vi "test Check UDP Properties and Redundancy.vi"(8 "error in":errorcluster, 11 "TestCase in":refnum<class "AIM ARINC 664 EncodeDecode.lvclass">) -> (0 "error out":errorcluster, 3 "TestCase out":refnum<class "AIM ARINC 664 EncodeDecode.lvclass">)   [LabVIEW 2020, in "AIM ARINC 664 EncodeDecode.lvclass"]
uses:
  AIM ARINC 664 EncodeDecode.lvclass
  C:/Program Files (x86)/National Instruments/LabVIEW 2020/vi.lib/NI/VeriStand Custom Device Testing Tools/VeriStandScriptingTestCase/VeriStandScriptingTestCase.lvclass
  Import/_typedefs/board_setup.ctl
  Import/_typedefs/tx_udp_setup.ctl
  Import/_typedefs/port_tx_udp_comm.ctl
  Import/_typedefs/frame_parameter.ctl
  Import/_typedefs/frame_parameter_definition.ctl
  <vilib>/NI/NI VeriStand Encoding and Decoding/Encoding.ctl
  Import/_typedefs/port_tx_udp_sap.ctl
  Import/_typedefs/rx_udp_setup.ctl
  Import/_typedefs/port_rx_udp_comm.ctl
  Import/_typedefs/port_rx_udp_sap.ctl
  <vilib>/NI/VeriStand Custom Device Testing Tools/VeriStandScriptingTestCase/VeriStandScriptingTestCase.lvclass/VeriStandScriptingTestCase.ctl
  <vilib>/NI/VeriStand Custom Device Testing Tools/VeriStandScriptingTestCase/Read Target.vi
  NationalInstruments.VeriStand.SystemDefinitionAPI
  <vilib>/addons/_JKI Toolkits/VI Tester/TestCase.llb/TestCase.lvclass
  Scripting/AIM ARINC 664 Scripting.lvlib
  Import/AIM ARINC 664 Import.lvlib
  <vilib>/NI/NI VeriStand Encoding and Decoding/Encoding and Decoding.lvlib
  C:/Program Files (x86)/National Instruments/LabVIEW 2020/vi.lib/addons/_JKI Toolkits/VI Tester/TestCase.llb/TestCase.lvclass
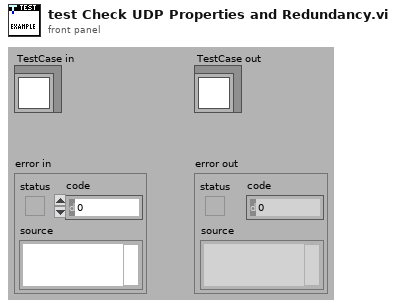
[diagram p1: front panel]
types:
  T1 = typedef "AIM ARINC 664 Import.lvlib/rx_udp_setup.ctl" = cluster{"VerificationMode":u32, "Bag":u32, "Jitter":u32, "MaxFrameLength":u32, "MaxSkew":u32, "VLBufSize":u32, "FilterMode":u32, "FilterPosition":u32, "Padding":u32, "FilterMask":u32, "FilterData":u32, "MinFrameLength":u32, "VlId":u16, "VLRange":u32}
  T2 = typedef "AIM ARINC 664 Import.lvlib/port_rx_udp_comm.ctl" = cluster{"PayloadID":string, "domainID":u8, "sideID":u8, "locationID":u8, "partitionID":u8, "UdpSrcPort":u16, "UdpDstPort":u16, "PortType":enum16{"FDX_UDP_SAMPLING", "FDX_UDP_QUEUING"}, "SubVIId":u32, "UdpNumBufMessages":u32, "UdpMaxMessageSize":u32, "UdpSamplingRate":u32, "Parameters":T3[]}
  T3 = typedef "AIM ARINC 664 Import.lvlib/frame_parameter.ctl" = cluster{"name":string, "default value":dbl, "unit":string, "Parameter":T4}
  T4 = typedef "AIM ARINC 664 Import.lvlib/frame_parameter_definition.ctl" = cluster{"start index":i32, "size":i32, "encoding":T5, "signed":bool, "scale multiplier":dbl, "scale offset":dbl}
  T5 = typedef "Encoding and Decoding.lvlib/Encoding.ctl" = enum16{"BNR", "BCD", "Discrete"}
  T6 = typedef "AIM ARINC 664 Import.lvlib/port_rx_udp_sap.ctl" = cluster{"PayloadID":string, "UdpDstPort":u16, "UdpNumBufMessages":u32, "UdpMaxMessageSize":u32, "Parameters":T3[]}
  T7 = cluster{"Tx_UDP":T1, "commPorts":T2[], "sapPorts":T6[]}[]
  T8 = typedef "AIM ARINC 664 Import.lvlib/tx_udp_setup.ctl" = cluster{"VlId":i32, "Bag":i32, "NetSelect":u32, "domainID":u8, "sideID":u8, "locationID":u8, "interfaceID":u8, "NumOfSubVl":u16, "Skew":u32, "MaxFrameLength":u32, "FrameBufferSize":u32}
  T9 = typedef "AIM ARINC 664 Import.lvlib/port_tx_udp_comm.ctl" = cluster{"PayloadID":string, "partitionID":u8, "UdpSrcPort":u16, "UdpDstPort":u16, "PortType":enum16{"FDX_UDP_SAMPLING", "FDX_UDP_QUEUING"}, "SubVIId":u32, "UdpNumBufMessages":u32, "UdpMaxMessageSize":u32, "UdpSamplingRate":u32, "Parameters":T3[]}
  T10 = typedef "AIM ARINC 664 Import.lvlib/port_tx_udp_sap.ctl" = cluster{"PayloadID":string, "SubVlId":u8, "UdpSrcPort":u16, "UdpNumBufMessages":u32, "UdpMaxMessageSize":u32, "partitionID":u8, "domainID":u8, "sideID":u8, "locationID":u8, "interfaceID":u8, "Parameters":T3[]}
  T11 = cluster{"tx_udp_setup":T8, "commPorts":T9[], "sapPorts":T10[]}[]
  T12 = typedef "AIM ARINC 664 Import.lvlib/board_setup.ctl" = cluster{"boardId":u32, "portSpeed":u32, "portConfig":u32}
  T13 = typedef "Custom Device API.lvlib/Custom Device Item Ref.ctl" = u64
  T14 = typedef "AIM ARINC 664 Import.lvlib/port_setup.ctl" = cluster{"port Id":u32, "redundant":bool}
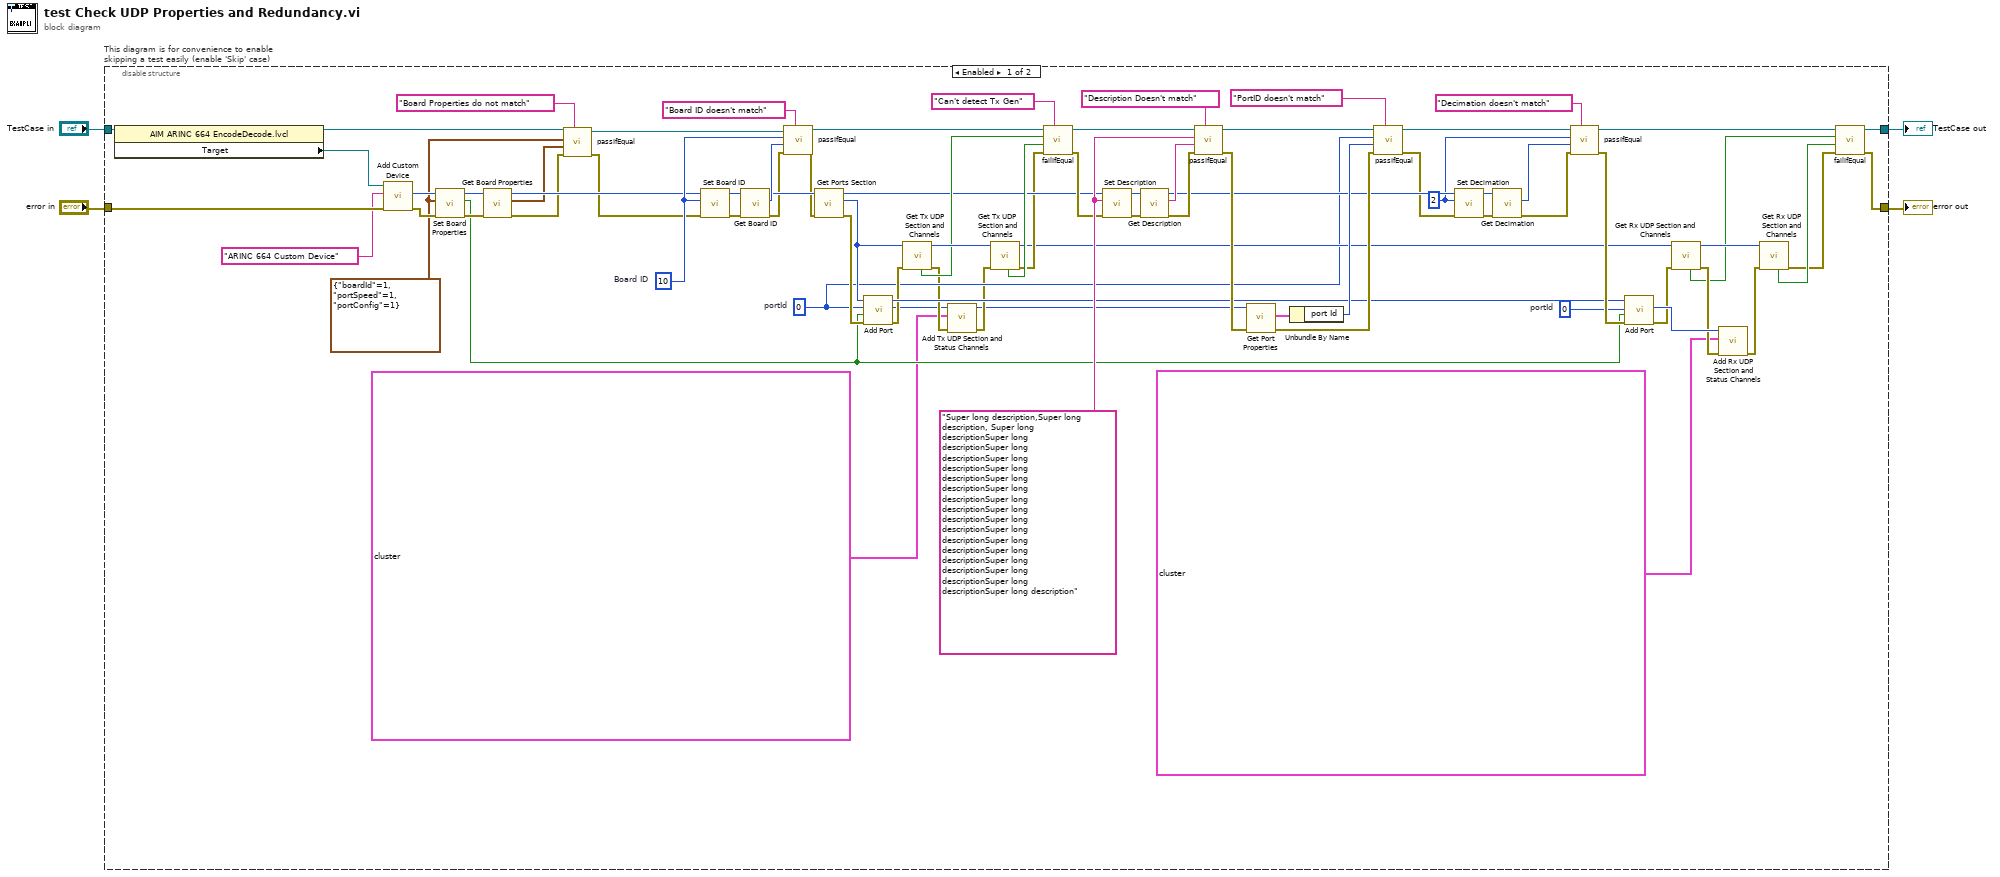
[diagram p0: block diagram]
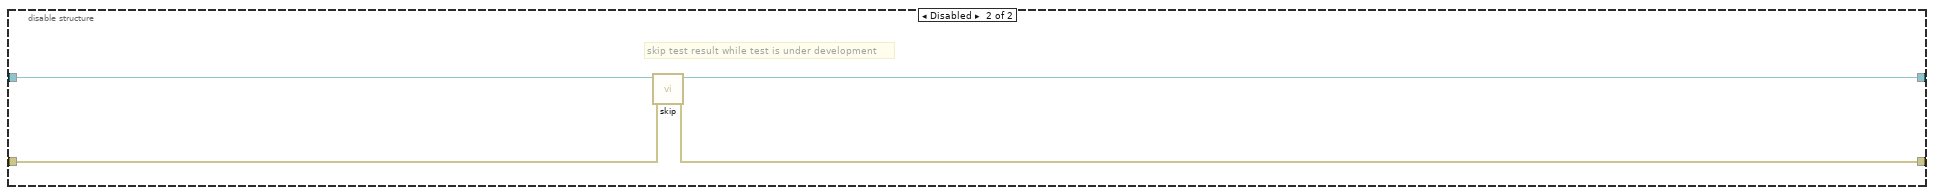
[diagram p2: hidden frame]
diagram:
  n1 = disable-structure "This diagram is for convenience to enable skipping a test easily (enable 'Skip' case)" shown="Enabled" {
    disable-tunnel: "TestCase in" -> [w83 w88]
    disable-tunnel: [w31 w86] -> w1
    disable-tunnel: [w27 w87] -> w3
    disable-tunnel: "error in" -> [w84 w85]
    frame Enabled {
      w17 = T12 {"boardId"=1, "portSpeed"=1, "portConfig"=1} ("board setup")
      w25 = u32 0  # portId
      w26 = u32 0  # portId
      w60 = 2 ("decimation")
      w77 = "Super long description,Super long description, Super long descriptionSuper long descriptionSuper long descriptionSuper long descriptionSuper long descriptionSuper long descriptionSuper long descriptionSuper long descriptionSuper long descriptionSuper long descriptionSuper long descriptionSuper long descriptionSuper long descriptionSuper long descriptionSuper long descriptionSuper long descriptionSuper long description" ("description")
      w69 = 10  # Board ID
      n2 = property class="AIM ARINC 664 EncodeDecode.lvcl"(reference=w83) -> (reference out=w16:refnum<class "AIM ARINC 664 EncodeDecode.lvclass">, "Target"=w82:refnum<k24>)  [unwired: 1 in, 1 out]
      n3 = call "Add Custom Device.vi"("error in"=w84, "name"="ARINC 664 Custom Device", "target in"=w82) -> ("error out"=w21:errorcluster, "custom device"=w23:T13)  [unwired: 6 in, 1 out]
      n4 = call "Set Board Properties.vi"("error in"=w21, "board setup"=w17, "custom device ref in"=w23) -> ("error out"=w20:errorcluster, "redundant?"=w19:bool, "custom device ref out"=w22:T13)  [unwired: 6 in]
      n5 = call "Get Board Properties.vi"("error in"=w20, "custom device ref"=w22) -> ("error out"=w14:errorcluster, "board properties out"=w11:T12, "custom device ref out"=w18:T13)  [unwired: 7 in]
      n6 = call-dynamic "passIfEqual.vi"("custom report message (\"\")"="Board Properties do not match" ("custom report message (\"\")"), "error in (no error)"=w14, "y"=w11, "x"=w17, "TestCase in"=w16) -> ("error out"=w13:errorcluster, "TestCase out"=w15:refnum<class "AIM ARINC 664 EncodeDecode.lvclass">)  [unwired: 5 in]
      n7 = call "Set Board ID.vi"("error in"=w13, "Board ID"=w69, "custom device ref"=w18) -> ("error out"=w50:errorcluster, "custom device ref out"=w51:T13)  [unwired: 7 in]
      n8 = call "Get Board ID.vi"("error in"=w50, "custom device ref"=w51) -> ("error out"=w48:errorcluster, "Board ID"=w70:i32, "custom device ref out"=w49:T13)  [unwired: 7 in]
      n9 = call-dynamic "passIfEqual.vi"("custom report message (\"\")"="Board ID doesn't match" ("description"), "error in (no error)"=w48, "y"=w70, "x"=w69, "TestCase in"=w15) -> ("error out"=w24:errorcluster, "TestCase out"=w47:refnum<class "AIM ARINC 664 EncodeDecode.lvclass">)  [unwired: 5 in]
      n10 = call "Get Ports Section.vi"("error in"=w24, "custom device ref"=w49) -> ("error out"=w80:errorcluster, "ports ref out"=w52:T13, "custom device ref out"=w40:T13)  [unwired: 6 in, 1 out]
      n11 = call "Add Port.vi"("error in"=w80, "redundant ?"=w19, "port Id"=w26, "ports ref"=w52) -> ("error out"=w53:errorcluster, "port ref out"=w8:T13, "ports ref out"=w55:T13)  [unwired: 5 in]
      n12 = call "Get Tx UDP Section and Channels.vi"("error in"=w53, "custom device ref in"=w52) -> ("error out"=w10:errorcluster, "custom device ref out"=w45:T13, "channels found?"=w44:bool)  [unwired: 4 in, 3 out]
      n13 = call "Add Tx UDP Section and Status Channels.vi"("error in"=w10, "Tx UDP configuration"=T11 [{"tx_udp_setup"={"VlId"=0, "Bag"=0, "NetSelect"=0, "domainID"=1, "sideID"=1, "locationID"=1, "interfaceID"=1, "NumOfSubVl"=0, "Skew"=0, "MaxFrameLength"=0, "FrameBufferSize"=0}, "commPorts"=[{"PayloadID"="", "partitionID"=1, "UdpSrcPort"=0, "UdpDstPort"=0, "PortType"=enum."FDX_UDP_SAMPLING", "SubVIId"=0, "UdpNumBufMessages"=0, "UdpMaxMessageSize"=0, "UdpSamplingRate"=0, "Parameters"=[]}], "sapPorts"=[]}], "port ref"=w8) -> ("error out"=w9:errorcluster, "port ref out"=w7:T13)  [unwired: 7 in]
      n14 = call "Get Tx UDP Section and Channels.vi"("error in"=w9, "custom device ref in"=w45) -> ("error out"=w39:errorcluster, "custom device ref out"=w37:T13, "channels found?"=w43:bool)  [unwired: 4 in, 3 out]
      n15 = call-dynamic "failIfEqual.vi"("custom report message (\"\")"="Can't detect Tx Gen" ("custom report message (\"\")"), "error in (no error)"=w39, "y"=w43, "x"=w44, "TestCase in"=w47) -> ("error out"=w42:errorcluster, "TestCase out"=w46:refnum<class "AIM ARINC 664 EncodeDecode.lvclass">)  [unwired: 5 in]
      n16 = call "Set Description.vi"("error in"=w42, "description"=w77, "custom device ref"=w40) -> ("error out"=w78:errorcluster, "custom device ref out"=w79:T13)  [unwired: 7 in]
      n17 = call "Get Description.vi"("error in"=w78, "custom device ref"=w79) -> ("error out"=w76:errorcluster, "description"=w68:string, "custom device ref out"=w64:T13)  [unwired: 7 in]
      n18 = call-dynamic "passIfEqual.vi"("custom report message (\"\")"="Description Doesn't match" ("custom report message (\"\")"), "error in (no error)"=w76, "y"=w68, "x"=w77, "TestCase in"=w46) -> ("error out"=w75:errorcluster, "TestCase out"=w73:refnum<class "AIM ARINC 664 EncodeDecode.lvclass">)  [unwired: 5 in]
      n19 = call "Get Port Properties.vi"("error in"=w75, "custom device ref"=w7) -> ("error out"=w71:errorcluster, "port properties out"=w74:T14)  [unwired: 7 in, 1 out]
      n20 = Unbundle By Name(w74) -> ("port Id"=w72:u32)
      n21 = call-dynamic "passIfEqual.vi"("custom report message (\"\")"="PortID doesn't match" ("description"), "error in (no error)"=w71, "y"=w72, "x"=w26, "TestCase in"=w73) -> ("error out"=w63:errorcluster, "TestCase out"=w57:refnum<class "AIM ARINC 664 EncodeDecode.lvclass">)  [unwired: 5 in]
      n22 = call "Set Decimation.vi"("error in"=w63, "decimation"=w60, "custom device ref"=w64) -> ("error out"=w62:errorcluster, "custom device ref out"=w59:T13)  [unwired: 7 in]
      n23 = call "Get Decimation.vi"("error in"=w62, "custom device ref"=w59) -> ("error out"=w61:errorcluster, "decimation"=w58:i32)  [unwired: 7 in, 1 out]
      n24 = call-dynamic "passIfEqual.vi"("custom report message (\"\")"="Decimation doesn't match" ("description"), "error in (no error)"=w61, "y"=w58, "x"=w60, "TestCase in"=w57) -> ("error out"=w56:errorcluster, "TestCase out"=w32:refnum<class "AIM ARINC 664 EncodeDecode.lvclass">)  [unwired: 5 in]
      n25 = call "Add Port.vi"("error in"=w56, "redundant ?"=w19, "port Id"=w25, "ports ref"=w55) -> ("error out"=w38:errorcluster, "port ref out"=w54:T13)  [unwired: 5 in, 1 out]
      n26 = call "Get Rx UDP Section and Channels.vi"("error in"=w38, "custom device ref in"=w37) -> ("error out"=w35:errorcluster, "custom device ref out"=w33:T13, "found?"=w30:bool)  [unwired: 5 in, 2 out]
      n27 = call "Add Rx UDP Section and Status Channels.vi"("error in"=w35, "Rx UDP configuration"=T7 [{"Tx_UDP"={"VerificationMode"=65535, "Bag"=0, "Jitter"=0, "MaxFrameLength"=0, "MaxSkew"=0, "VLBufSize"=32768, "FilterMode"=0, "FilterPosition"=0, "Padding"=0, "FilterMask"=0, "FilterData"=0, "MinFrameLength"=0, "VlId"=0, "VLRange"=0}, "commPorts"=[{"PayloadID"="", "domainID"=0, "sideID"=0, "locationID"=0, "partitionID"=0, "UdpSrcPort"=0, "UdpDstPort"=0, "PortType"=enum."FDX_UDP_SAMPLING", "SubVIId"=0, "UdpNumBufMessages"=1, "UdpMaxMessageSize"=0, "UdpSamplingRate"=0, "Parameters"=[]}], "sapPorts"=[]}], "port ref"=w54) -> ("error out"=w34:errorcluster)  [unwired: 7 in, 1 out]
      n28 = call "Get Rx UDP Section and Channels.vi"("error in"=w34, "custom device ref in"=w33) -> ("error out"=w28:errorcluster, "found?"=w29:bool)  [unwired: 5 in, 3 out]
      n29 = call-dynamic "failIfEqual.vi"("error in (no error)"=w28, "y"=w29, "x"=w30, "TestCase in"=w32) -> ("error out"=w27:errorcluster, "TestCase out"=w31:refnum<class "AIM ARINC 664 EncodeDecode.lvclass">)  [unwired: 6 in]
    }
    frame Disabled {
      # "skip test result while test is under development"
      n30 = call <vilib>:"skip.vi"("error in (no error)"=w85, "TestCase in"=w88) -> ("error out"=w87:errorcluster, "TestCase out"=w86:refnum<class "AIM ARINC 664 EncodeDecode.lvclass">)  [unwired: 8 in]
    }
  }
  "error out" <- w3
  "TestCase out" <- w1
